vi "Plink example.vi"(6 "log file name":string="Log_filename", 7 "Verbose(f)":bool, 8 "error in (no error)":errorcluster, 9 "Password":string="Password", 10 "script filename":path, 11 "Saved Session":string="session_name") -> (0 "error out":errorcluster)   [LabVIEW 2016]
uses:
  <vilib>/Utility/sysdir.llb/System Directory Type.ctl
panel:
  out "Log file lines":string[](array[string])
  out "Command line":string
  out "Log file contents":string
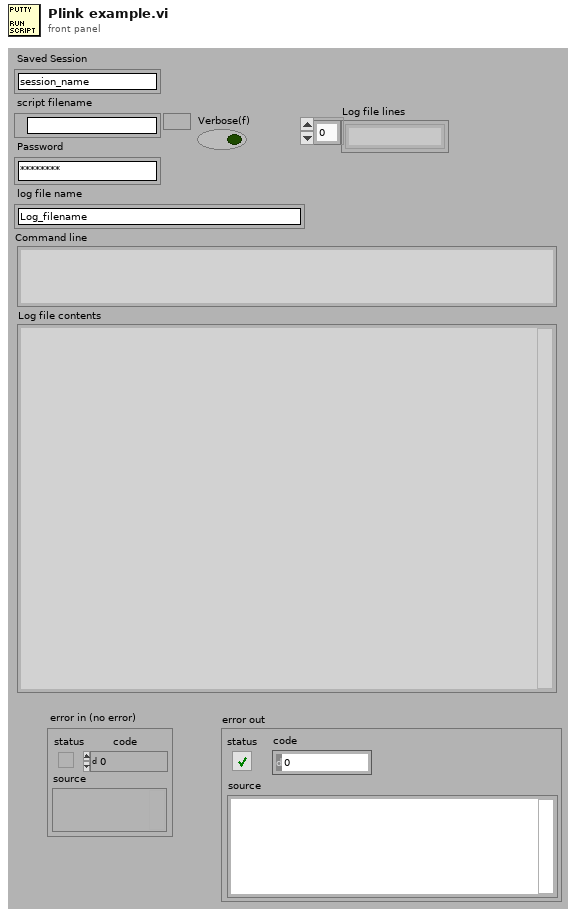
[diagram p1: front panel]
types:
  T1 = typedef "System Directory Type.ctl" = i32
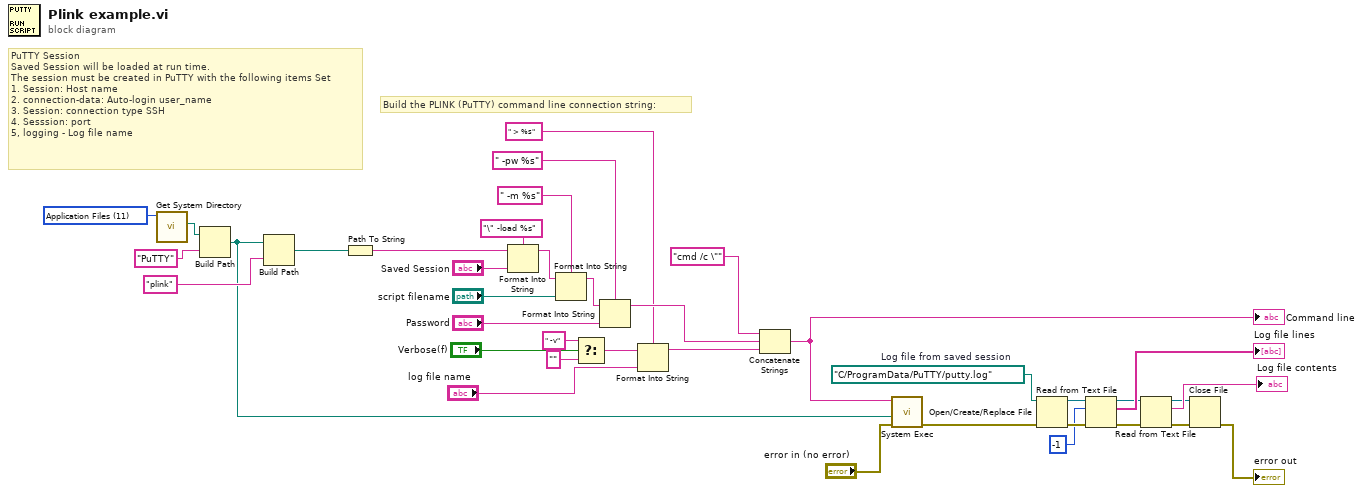
[diagram p0: block diagram]
diagram:
  w36 = path "C:/ProgramData/PuTTY/putty.log"  # Log file from saved session
  w38 = T1 11 items=["User Home"=0, "User Desktop"=1, "User Documents"=2, "User Application Data"=3, "User Preferences"=4, "User Temporary"=5, "Public Documents"=6, "Public Application Data"=7, "Public Preferences"=8, "Public Cache"=13, "System Core Libraries"=9, "System Installed Libraries"=10, "Application Files"=11, "Boot Volume Root"=12] ("system directory type")
  # "PuTTY Session\nSaved Session will be loaded at run time.\nThe session must be created in PuTTY with the following items Set\n1. Session: Host name\n2. connection-data: Auto-login user_name\n3. Session: connection type SSH\n4. Sesssion: port\n5, logging - Log file name"
  # "Build the PLINK (PuTTY) command line connection string:"
  n1 = call <vilib>:"Get System Directory.vi"("system directory type"=w38) -> ("system directory"=w33:path)  [unwired: 10 in]
  n2 = Build Path(base path=w33, name or relative path="PuTTY") -> (appended path=w30:path)
  n3 = Build Path(base path=w30, name or relative path="plink") -> (appended path=w1:path)
  n4 = Path To String(path=w1) -> (string=w6:string)
  n5 = Format Into String(format string="\" -load %s" ("name or relative path"), initial string=w6, "Saved Session") -> (resulting string=w8:string)  [unwired: 1 in, 1 out]
  n6 = Format Into String(format string=" -m %s" ("name or relative path"), initial string=w8, "script filename") -> (resulting string=w9:string)  [unwired: 1 in, 1 out]
  n7 = Select(t=" -v" ("name or relative path"), s="Verbose(f)", f="") -> (s? t:f=w7:string)
  n8 = Format Into String(format string=" -pw %s" ("name or relative path"), initial string=w9, "Password") -> (resulting string=w17:string)  [unwired: 1 in, 1 out]
  n9 = Format Into String(format string=" > %s" ("name or relative path"), initial string=w7, "log file name") -> (resulting string=w12:string)  [unwired: 1 in, 1 out]
  n10 = Concatenate Strings("cmd /c \"" ("name or relative path"), w17, w12) -> (w23:string)
  "Command line" <- w23
  n11 = call <vilib>:"System Exec.vi"("error in (no error)"="error in (no error)", "working directory"=w30, "command line"=w23) -> ("error out"=w2:errorcluster)  [unwired: 5 in, 3 out]
  n12 = Open/Create/Replace File(file path (use dialog)=w36, error in=w2) -> (refnum out=w27:refnum<file>, error out=w37:errorcluster)  [unwired: 4 in, 1 out]
  n13 = Read from Text File(file (use dialog)=w27, count=-1, error in=w37) -> (refnum out=w4:refnum<file>, text=→"Log file lines":string[], error out=w26:errorcluster)  [unwired: 1 in, 1 out]
  n14 = Read from Text File(file (use dialog)=w4, error in=w26) -> (refnum out=w3:refnum<file>, text=→"Log file contents":string, error out=w25:errorcluster)  [unwired: 2 in, 1 out]
  n15 = Close File(refnum=w3, error in=w25) -> (error out=→"error out":errorcluster)  [unwired: 1 out]
